vi "test Calculate Temperature Change-Change ra10 rte20 ate30 i0.1 sht.vi"(8 "error in (no error)":errorcluster, 11 "TestCase in":refnum<class "Calculate Temperature Change.lvclass">) -> (0 "error out":errorcluster, 3 "TestCase out":refnum<class "Calculate Temperature Change.lvclass">)   [LabVIEW 2018, in "Calculate Temperature Change.lvclass"]
uses:
  Calculate Temperature Change.lvclass
  Libraries/Thermal Chamber Response Simulator/Thermal Chamber Response Simulator.lvlib
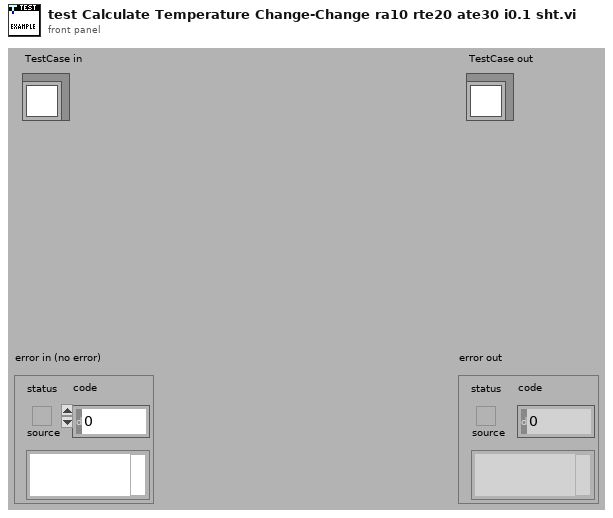
[diagram p1: front panel]
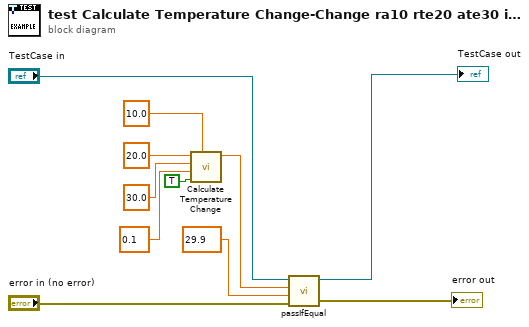
[diagram p0: block diagram]
diagram:
  n1 = call "Calculate Temperature Change.vi"("Ramp Rate deg C/s"=10.0, "Shutdown"=TRUE, "Time Interval (s)"=0.1, "Actual Temperature in deg C"=30.0, "Required Temperature deg C"=20.0) -> ("Actual Temperature out"=w6:dbl)  [unwired: 6 in]
  n2 = call-dynamic "passIfEqual.vi"("error in (no error)"="error in (no error)", "y"=29.9 ("Actual Temperature out"), "x"=w6, "TestCase in"="TestCase in") -> ("error out"=→"error out":errorcluster, "TestCase out"=→"TestCase out":refnum<class "Calculate Temperature Change.lvclass">)  [unwired: 6 in]
